vi "GetZeroIndex.vi"(11 "fft cluster":T1) -> (1 "Nx/2+1":dbl, 3 "Ny/2+1":dbl)   [LabVIEW 2018, in "myFFT.lvlib"]
uses:
  myFFT.lvlib
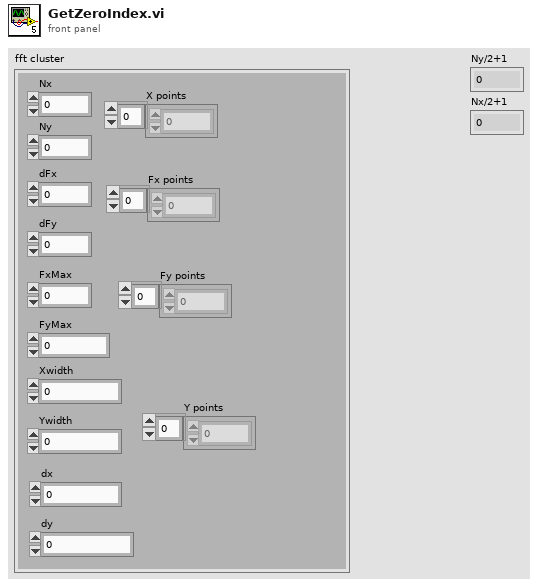
[diagram p1: front panel]
types:
  T1 = cluster{"dFx":dbl, "dFy":dbl, "Nx":i32, "Ny":i32, "FxMax":dbl, "FyMax":dbl, "Xwidth":dbl, "Ywidth":dbl, "dx":dbl, "dy":dbl, "Fx points":dbl[], "X points":dbl[], "Y points":dbl[], "Fy points":dbl[]}
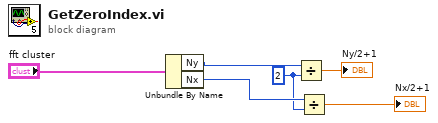
[diagram p0: block diagram]
diagram:
  w4 = 2 ("y")
  n1 = Unbundle By Name("fft cluster") -> ("Ny"=w3:i32, "Nx"=w5:i32)
  n2 = Divide(x=w3, y=w4) -> (x/y=→"Ny/2+1":dbl)
  n3 = Divide(x=w5, y=w4) -> (x/y=→"Nx/2+1":dbl)
